vi "Apply.vi"(8 "error in (no error)":errorcluster, 11 "DIO DAQmx PWM CFG in":refnum<class "CO DAQmx PWM CFG.lvclass">) -> (0 "error out":errorcluster, 3 "DIO DAQmx PWM CFG out":refnum<class "CO DAQmx PWM CFG.lvclass">)   [LabVIEW 2023, in "DAQmx Simulated CFGs.lvlib" / "CO DAQmx PWM CFG.lvclass"]
uses:
  CO DAQmx PWM CFG.lvclass
  Configuration/Configuration JSON/Configuration JSON Base/CFG JSON.lvclass/CFG JSON.ctl
  CO DAQmx PWM CFG/CO DAQmx PWM CFG.lvclass
  CO DAQmx PWM CFG.lvclass/CO DAQmx PWM CFG.ctl
  Configuration/Configuration JSON/Configuration JSON Base/CFG JSON.lvclass
  D:/git/HAL/HAL GOOP4/DIO/CO DAQmx PWM CFG/CO DAQmx PWM CFG.lvclass
  D:/git/HAL/HAL GOOP4/DAQmx/DAQmx Base CFG/DAQmx Base CFG.lvclass
  D:/git/HAL/HAL GOOP4/CFG Target/CFG Target.lvclass
  D:/git/HAL/HAL GOOP4/Configuration/Configuration Semaphore/CFG Semaphore.lvclass
  D:/git/HAL/HAL GOOP4/Configuration/Configuration JSON/Configuration JSON Base/CFG JSON.lvclass
  D:/git/HAL/HAL GOOP4/Interfaces/IConfigure/IConfigure.lvclass
  D:/git/HAL/HAL GOOP4/DIO/DIO DAQmx Simulated CFGs/CO DAQmx PWM CFG/CO DAQmx PWM CFG.lvclass
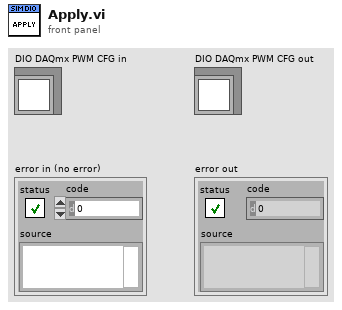
[diagram p1: front panel]
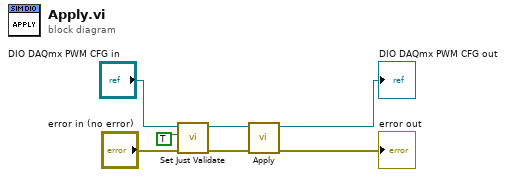
[diagram p0: block diagram]
diagram:
  n1 = call "Set Just Validate.vi"("error in (no error)"="error in (no error)", "Just Validate"=TRUE, "CFG JSON Base in"="DIO DAQmx PWM CFG in") -> ("error out"=w4:errorcluster, "CFG JSON Base out"=w2:refnum<class "CO DAQmx PWM CFG.lvclass">)  [unwired: 7 in]
  n2 = call-parent "Apply.vi"("error in (no error)"=w4, "DIO DAQmx PWM CFG in"=w2) -> ("error out"=→"error out":errorcluster, "DIO DAQmx PWM CFG out"=→"DIO DAQmx PWM CFG out":refnum<class "CO DAQmx PWM CFG.lvclass">)  [unwired: 8 in]
